vi "Initialise.vi"(8 "error in (no error)":errorcluster, 10 "Message in":refnum<class "InitialiseMessage.lvclass">, 11 "DAQCascade512II in":refnum<class "DAQCascade512II.lvclass">) -> (0 "error out":errorcluster, 3 "DAQCascade512II out":refnum<class "DAQCascade512II.lvclass">)   [LabVIEW 2012, in "DAQCascade512II.lvclass"]
doc: "This method is called when an initialise message is received. It mainly initialises the RabbitMQ connectivity. \n\nOverride this method when your component needs special initialisation (e.g. of software or hardware resources). In that case, don't forget to call the parent for proper implementation. If your component owns subcomponents, they count as resources, so you have to initialise them by calling their own initialise functions"
uses:
  DAQCascade512II.lvclass
  <vilib>/Distrio/Murmex/InitialiseMessage/InitialiseMessage.lvclass
  <vilib>/Distrio/Murmex/Murmex/Murmex.lvclass
  DAQCascade512II.lvclass/DAQCascade512II.ctl
panel:
  out "intialized?":bool
  # "This method is called when the INTIALISE\ntrigger is sent. \n\nOverride this method when your component needs to\nrespond to this trigger. \n\nCall parent for proper implementation"
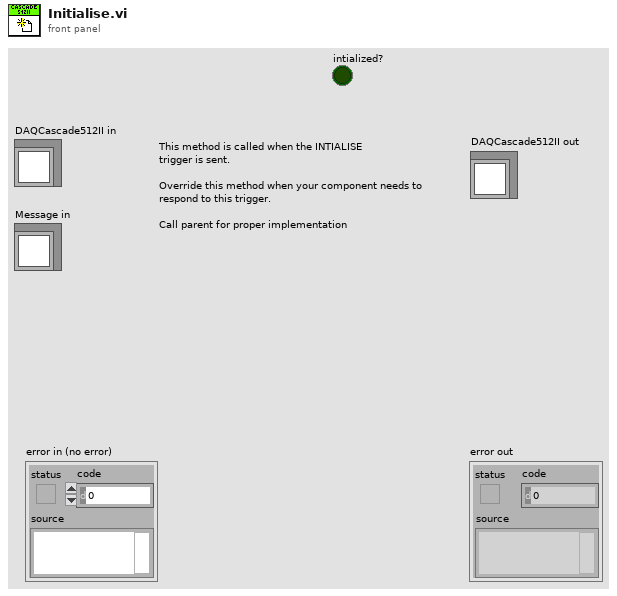
[diagram p1: front panel]
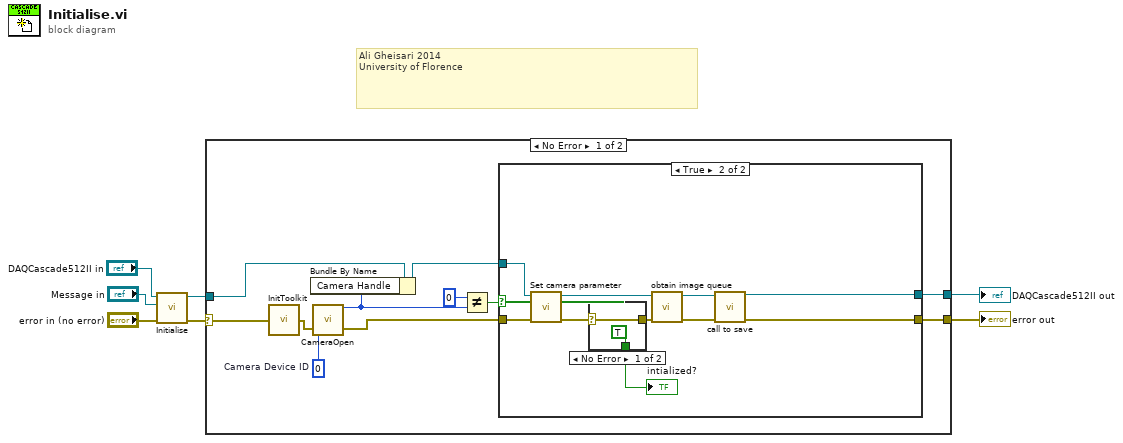
[diagram p0: block diagram]
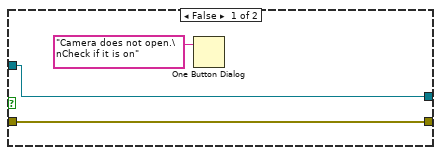
[diagram p2: hidden frame]
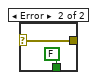
[diagram p3: hidden frame]
diagram:
  # "Ali Gheisari 2014\nUniversity of Florence"
  n1 = call-parent "Initialise.vi"("error in (no error)"="error in (no error)", "Message in"="Message in", "Murmex in"="DAQCascade512II in") -> ("error out"=w4:errorcluster, "Murmex out"=w2:refnum<class "DAQCascade512II.lvclass">)  [unwired: 7 in]
  n2 = case shown="No Error" w4 {
    selector: w4 -> [w18 w37]
    tunnel: [w14 w37] -> w3
    tunnel: [w15 w36] -> w1
    tunnel: w2 -> [w10 w36]
    frame No Error {
      w17 = u32 0  # Camera Device ID
      n3 = call <userlib>:"InitToolkit.vi"("error in"=w18) -> ("error out"=w16:errorcluster)
      n4 = call <userlib>:"CameraOpen.vi"("error in"=w16, "Camera Device ID"=w17) -> ("error out"=w13:errorcluster, "Camera Handle"=w8:u32)
      n5 = Bundle By Name(cluster=w10, "Camera Handle"=w8) -> (w9:refnum<class "DAQCascade512II.lvclass">)
      n6 = Not Equal?(x=u32 0, y=w8) -> (x != y?=w11:bool)
      n7 = case shown="True" w11 {
        tunnel: w13 -> [w20 w30]
        tunnel: [w20 w22] -> w14
        tunnel: [w21 w24] -> w15
        tunnel: w9 -> [w21 w31]
        frame False {
          n8 = One Button Dialog(message="Camera does not open.\nCheck if it is on") -> ()  [unwired: 1 in, 1 out]
        }
        frame True {
          n9 = call-dynamic "Set camera parameter.vi"("error in (no error)"=w30, "DAQCascade512II in"=w31) -> ("error out"=w29:errorcluster, "DAQCascade512II out"=w26:refnum<class "DAQCascade512II.lvclass">)  [unwired: 8 in]
          n10 = case shown="No Error" w29 {
            selector: w29 -> [w32 w34]
            tunnel: [TRUE FALSE] -> w28
            tunnel: [w32 w34] -> w27
            frame No Error {
            }
            frame Error {
            }
          }
          "intialized?" <- w28
          n11 = call-dynamic "obtain image queue.vi"("error in (no error)"=w27, "DAQCascade512II in"=w26) -> ("error out"=w25:errorcluster, "DAQCascade512II out"=w23:refnum<class "DAQCascade512II.lvclass">)  [unwired: 8 in]
          n12 = call-dynamic "call to save.vi"("error in"=w25, "DAQCascade512II"=w23) -> ("error out"=w22:errorcluster, "DAQCascade512II out"=w24:refnum<class "DAQCascade512II.lvclass">)  [unwired: 8 in]
        }
      }
    }
    frame Error {
    }
  }
  "error out" <- w3
  "DAQCascade512II out" <- w1
